vi "gainsGlobalBot.vi"() -> ()   [LabVIEW 2013]
panel:
  in  "gains":T1
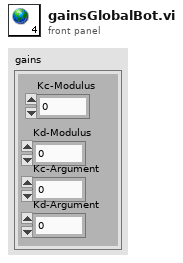
[diagram p1: front panel]
types:
  T1 = cluster{"Kc-Modulus":dbl, "Kd-Modulus":dbl, "Kc-Argument":dbl, "Kd-Argument":dbl}
diagram:
